vi "entrer daq.vi"() -> (0 "Tableau":dbl[](array[numeric]), 1 "vent":dbl, 3 "codeur":i32, 4 "pluie":bool)   [LabVIEW 2017]
uses:
  <vilib>/DAQmx/read.llb/DAQmx Read (Counter DBL 1Chan 1Samp).vi
  <vilib>/DAQmx/read.llb/DAQmx Read (Digital U8 1Chan 1Samp).vi
  <vilib>/DAQmx/read.llb/DAQmx Read (Digital Bool 1Line 1Point).vi
  <vilib>/DAQmx/read.llb/DAQmx Read (Analog 1D DBL NChan 1Samp).vi
  <vilib>/DAQmx/create/channels.llb/DAQmx Create Channel (AI-Voltage-Basic).vi
  <vilib>/DAQmx/miscellaneous.llb/DAQmx Fill In Error Info.vi
  <vilib>/DAQmx/create/channels.llb/DAQmx Create Channel (DI-Digital Input).vi
  <vilib>/DAQmx/create/channels.llb/DAQmx Create Channel (CI-Count Edges).vi
  <resource>/objmgr/daqmx.rc
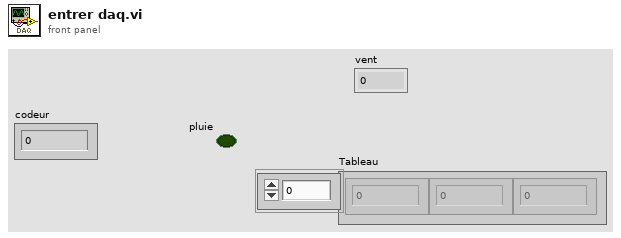
[diagram p1: front panel]
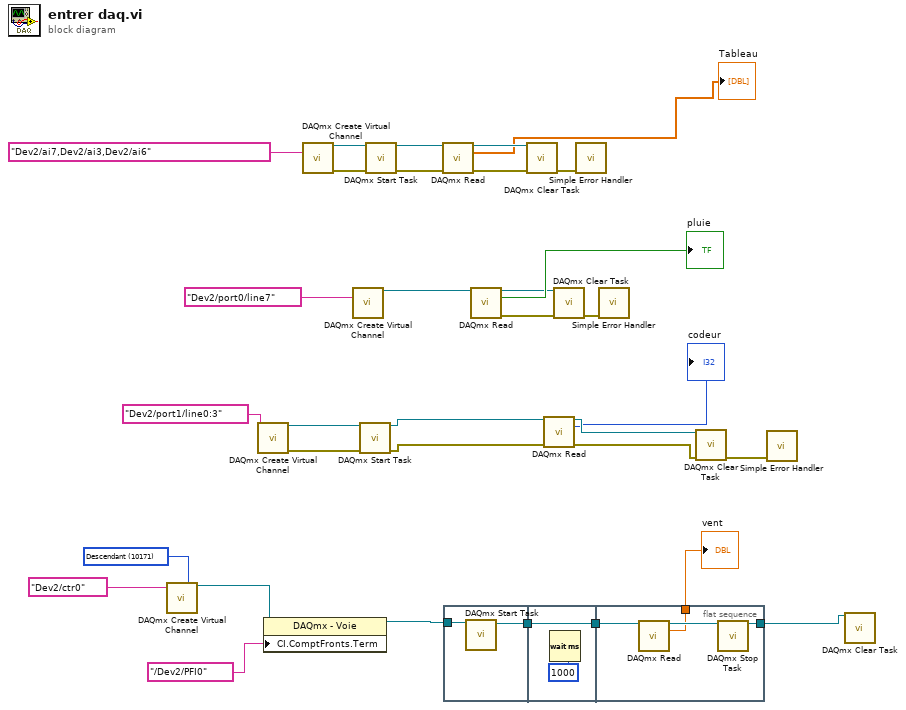
[diagram p0: block diagram]
diagram:
  w3 = 10171 items=["Montant"=10280, "Descendant"=10171] ("edge")
  n1 = call-poly <vilib>:"DAQmx Create Virtual Channel.vi"("edge"=w3, "counter"=tag "Dev2/ctr0") -> ("task out"=w5:refnum<k21>)  [unwired: 12 in, 1 out]
  n2 = call-poly <vilib>:"DAQmx Create Virtual Channel.vi"("lines"=tag "Dev2/port1/line0:3") -> ("task out"=w14:refnum<k21>, "error out"=w13:errorcluster)  [unwired: 13 in]
  n3 = property class="DAQmx - Voie"(reference=w5, "CI.ComptFronts.Term"=tag "/Dev2/PFI0" ("Démarr.FrontNum.Src")) -> (reference out=w7:refnum<k21>)  [unwired: 1 in, 1 out]
  n4 = call-poly <vilib>:"DAQmx Create Virtual Channel.vi"("physical channels"=tag "Dev2/ai7,Dev2/ai3,Dev2/ai6") -> ("task out"=w28:refnum<k21>, "error out"=w27:errorcluster)  [unwired: 13 in]
  n5 = call-poly <vilib>:"DAQmx Create Virtual Channel.vi"("lines"=tag "Dev2/port0/line7") -> ("task out"=w23:refnum<k21>)  [unwired: 13 in, 1 out]
  n6 = call <vilib>:"DAQmx Start Task.vi"("task/channels in"=w14, "error in"=w13) -> ("task out"=w16:refnum<k21>, "error out"=w17:errorcluster)  [unwired: 12 in]
  n7 = call <vilib>:"DAQmx Start Task.vi"("task/channels in"=w28, "error in"=w27) -> ("task out"=w29:refnum<k21>, "error out"=w30:errorcluster)  [unwired: 12 in]
  n8 = call-poly <vilib>:"DAQmx Read.vi"("task/channels in"=w29, "error in"=w30) -> ("task out"=w32:refnum<k21>, "data"=→"Tableau":dbl[], "error out"=w33:errorcluster)  [unwired: 11 in]
  n9 = flat-sequence {
    tunnel: w7 -> [w35]
    tunnel: [w34] -> w11
    tunnel: w11 -> [w36]
    tunnel: [w36] -> w10
    tunnel: w10 -> [w41]
    tunnel: [w39] -> w8
    tunnel: [w38] -> w9
    frame #0 {
      n10 = call <vilib>:"DAQmx Start Task.vi"("task/channels in"=w35) -> ("task out"=w34:refnum<k21>)  [unwired: 13 in, 1 out]
    }
    frame #1 {
      n11 = Wait (ms)(milliseconds to wait=u32 1000 ("attente (ms)")) -> ()  [unwired: 1 out]
    }
    frame #2 {
      n12 = call-poly <vilib>:"DAQmx Read.vi"("task/channels in"=w41) -> ("task out"=w40:refnum<k21>, "data"=w38:dbl)  [unwired: 12 in, 1 out]
      n13 = call <vilib>:"DAQmx Stop Task.vi"("task/channels in"=w40) -> ("task out"=w39:refnum<k21>)  [unwired: 13 in, 1 out]
    }
  }
  n14 = call-poly <vilib>:"DAQmx Read.vi"("task/channels in"=w23) -> ("task out"=w25:refnum<k21>, "data"=→"pluie":bool, "error out"=w24:errorcluster)  [unwired: 12 in]
  n15 = call <vilib>:"DAQmx Clear Task.vi"("task in"=w32, "error in"=w33) -> ("error out"=w31:errorcluster)  [unwired: 13 in]
  n16 = call-poly <vilib>:"DAQmx Read.vi"("task/channels in"=w16, "error in"=w17) -> ("task out"=w19:refnum<k21>, "data"=→"codeur":u8, "error out"=w20:errorcluster)  [unwired: 11 in]
  n17 = call <vilib>:"DAQmx Clear Task.vi"("task in"=w25, "error in"=w24) -> ("error out"=w21:errorcluster)  [unwired: 13 in]
  n18 = call <vilib>:"Simple Error Handler.vi"("error in (no error)"=w31) -> ()  [unwired: 4 in, 5 out]
  n19 = call <vilib>:"Simple Error Handler.vi"("error in (no error)"=w21) -> ()  [unwired: 4 in, 5 out]
  n20 = call <vilib>:"DAQmx Clear Task.vi"("task in"=w19, "error in"=w20) -> ("error out"=w18:errorcluster)  [unwired: 13 in]
  n21 = call <vilib>:"Simple Error Handler.vi"("error in (no error)"=w18) -> ()  [unwired: 4 in, 5 out]
  n22 = call <vilib>:"DAQmx Clear Task.vi"("task in"=w8) -> ()  [unwired: 14 in, 1 out]
  "vent" <- w9
